vi "WaitMeasure.vi"() -> ()   [LabVIEW 2018]
panel:
  out "显示":string="测量中"
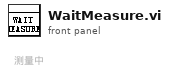
[diagram p1: front panel]
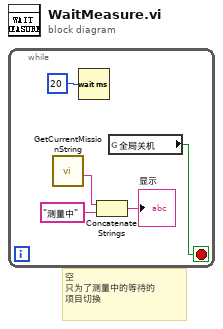
[diagram p0: block diagram]
diagram:
  # "空\n只为了测量中的等待的\n项目切换"
  n1 = while {
    stop <- w5 stop-if-true
    n2 = call "GetCurrentMissionString.vi"() -> ("任务字符串"=w3:string)  [unwired: 11 in]
    n3 = Wait (ms)(milliseconds to wait=u32 20 ("等待时间（毫秒）")) -> ()  [unwired: 1 out]
    n4 = Concatenate Strings(w3, "测量中" ("字符串")) -> (→"显示":string)
    n5 = global read "参数.vi" "全局关机"() -> (w5:bool)
  }
